vi "State_Machine.vi"(8 "error in (no error)":errorcluster caption="entrée d'erreur (pas d'erreur)", 11 "Get_Voltage en entrée":refnum<class "P2056_Set_SN_PCBA.lvclass">) -> (0 "error out":errorcluster caption="sortie d'erreur", 2 "Json_String":string, 3 "Get_Voltage en sortie":refnum<class "P2056_Set_SN_PCBA.lvclass">)   [LabVIEW 2020, in "Library Test.lvlib" / "P2056_Set_SN_PCBA.lvclass"]
uses:
  P2056_Set_SN_PCBA.lvclass
  C:/Users/ngarcin/OneDrive - Altyor/Standard TB/Suite TB45/Class/Test/P2056_Send_Command_UART/P2056_Send_Command_UART.lvclass
  Commun VI/TypeDef/Variable Printable.ctl
  P2056_Send_Command_UART.lvclass
  Commun VI/Library Commun.lvlib
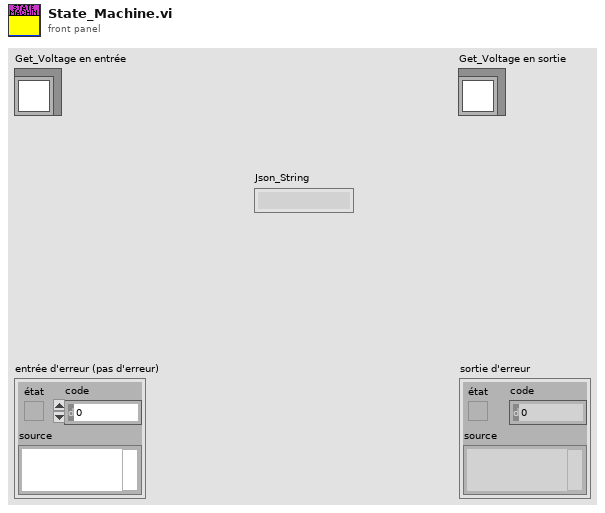
[diagram p1: front panel]
types:
  T1 = typedef "Variable Printable.ctl" = string
  T2 = enum16{"Get Variable", "Get All Variables", "Set Variable", "Delete Variable", "Delete All Variable"}
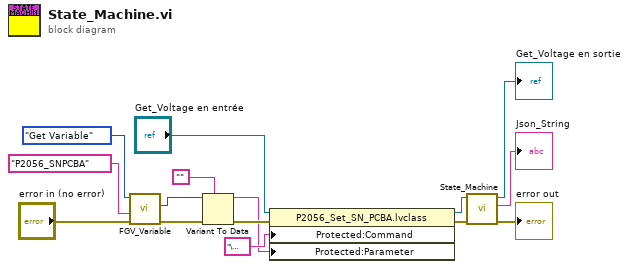
[diagram p0: block diagram]
diagram:
  n1 = call "FGV_Variable.vi"("error in (no error)"="error in (no error)", "Variable"=T1 "P2056_SNPCBA", "Function"=T2."Get Variable") -> ("error out"=w7:errorcluster, "Data Out"=w6:variant)  [unwired: 6 in, 1 out]
  n2 = Variant To Data(error in=w7, type="", Variant=w6) -> (data=w1:string, error out=w3:errorcluster)
  n3 = property class="P2056_Set_SN_PCBA.lvclass"(reference="Get_Voltage en entrée", error in=w3, "Protected:Command"="\u0013" ("chaîne"), "Protected:Parameter"=w1) -> (reference out=w13:refnum<class "P2056_Set_SN_PCBA.lvclass">, error out=w12:errorcluster)
  n4 = call-parent "State_Machine.vi"("error in (no error)"=w12, "Get_Voltage en entrée"=w13) -> ("error out"=→"error out":errorcluster, "Json_String"=→"Json_String":string, "Get_Voltage en sortie"=→"Get_Voltage en sortie":refnum<class "P2056_Set_SN_PCBA.lvclass">)  [unwired: 7 in]
